vi "Embedded UI.TestLauncher.vi"() -> ()   [LabVIEW 2019, in "Embedded UI.lvclass"]
doc: "JKI State Machine Objects (SMO) 1.0.0.5\nJKI - JKI\nCopyright (c) 2016, JKI"
uses:
  Embedded UI.lvclass
  <vilib>/JKI/JKI SMO/SMO/SMO.lvclass
  <vilib>/JKI/JKI SMO/SMO.UI/SMO.UI.lvclass
  <vilib>/JKI/JKI SMO/SMO/Typedefs/SMOState --Enum.ctl
  C:/Program Files (x86)/National Instruments/LabVIEW 2019/vi.lib/JKI/JKI SMO/SMO.UI/SMO.UI.lvclass
  C:/Program Files (x86)/National Instruments/LabVIEW 2019/vi.lib/JKI/JKI SMO/SMO/SMO.lvclass
panel:
  in  "Change Name":bool
  out "Get Name":string
  in  "Set Name":string
  in  "Embed?":bool
  out "error out":errorcluster
  in  "Stop":bool
  # "SMO UI Test Launcher"
  # "For instructions on how to use the JKI State Machine Objects, examples and video tutorials, visit:\nhttp://jki.net/state-machine-objects/\n\nJKI State Machine Objects™\nhttp://jki.net/state-machine-objects/\nCopyright (C) 2005-2015, JKI <info@jki.net>\nALL RIGHTS RESERVED"
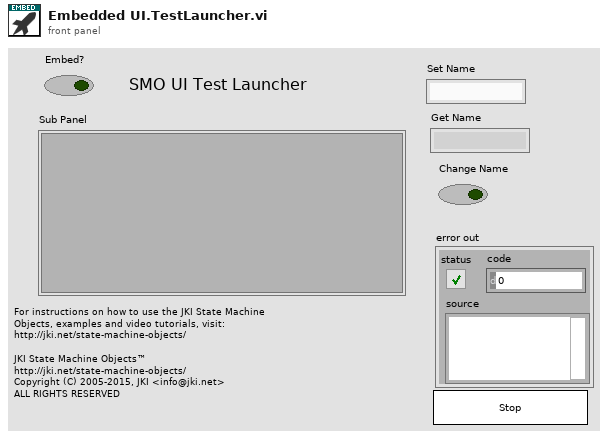
[diagram p1: front panel]
types:
  T1 = typedef "SMO.lvclass/Public Events.ctl" = cluster{"Error":refnum<user-event>, "State":refnum<user-event>, "Reserve State":refnum<user-event>}
  T2 = typedef "SMO.UI.lvclass/PublicEvents--Cluster.ctl" = cluster{"UI Hidden":refnum<user-event>, "UI State":refnum<user-event>}
  T3 = typedef "SMO.lvclass/SMOState --Enum.ctl" = enum16{"unknown", "Created", "Started", "Stopped"}
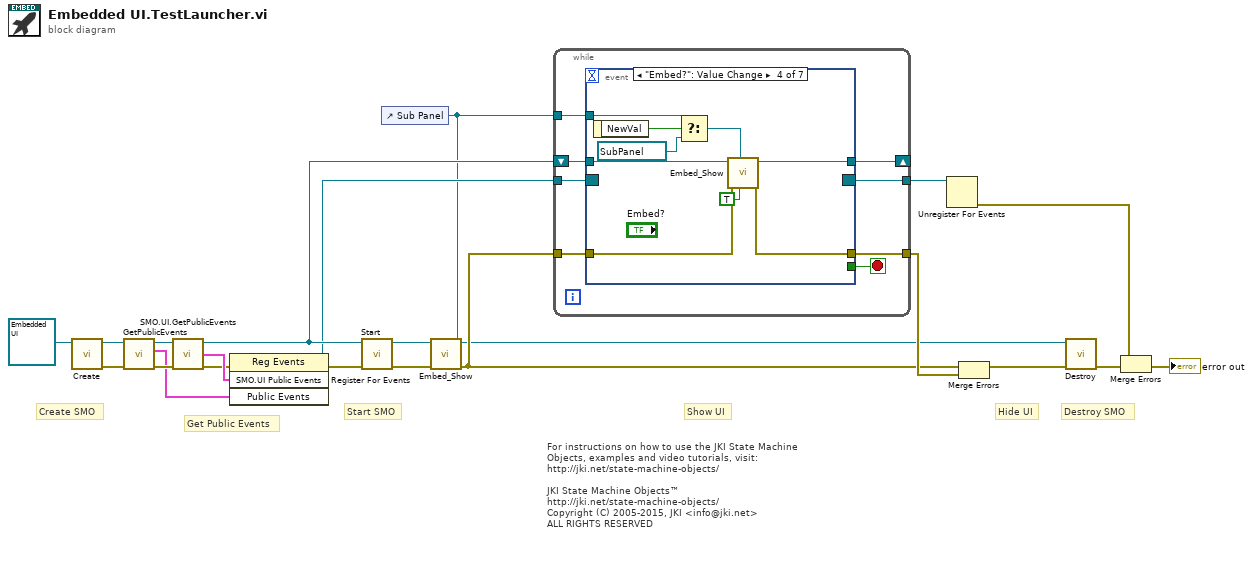
[diagram p0: block diagram]
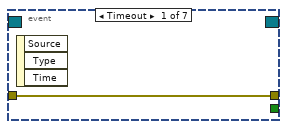
[diagram p2: hidden frame]
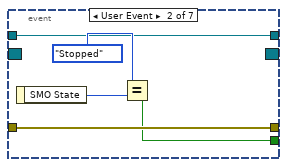
[diagram p3: hidden frame]
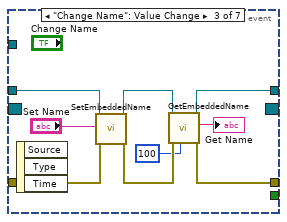
[diagram p4: hidden frame]
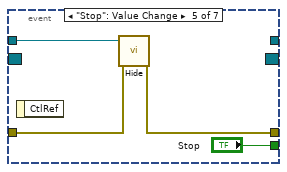
[diagram p5: hidden frame]
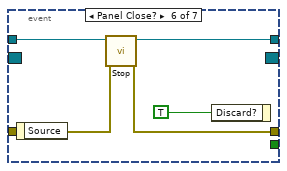
[diagram p6: hidden frame]
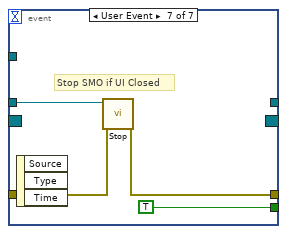
[diagram p7: hidden frame]
diagram:
  # "Hide UI"
  # "Show UI"
  # "For instructions on how to use the JKI State Machine Objects, examples and video tutorials, visit:\nhttp://jki.net/state-machine-objects/\n\nJKI State Machine Objects™\nhttp://jki.net/state-machine-objects/\nCopyright (C) 2005-2015, JKI <info@jki.net>\nALL RIGHTS RESERVED"
  # "Get Public Events"
  # "Start SMO"
  # "Destroy SMO"
  # "Create SMO"
  n1 = call <vilib>:"Create.vi"("SMO"=refnum<class "Embedded UI.lvclass"> refnum ("SMO.Template.lvclass")) -> ("error out"=w10:errorcluster, "SMO out"=w9:refnum<class "Embedded UI.lvclass">)  [unwired: 8 in, 1 out]
  n2 = call <vilib>:"GetPublicEvents.vi"("error in (no error)"=w10, "SMO"=w9) -> ("error out"=w7:errorcluster, "Public Events"=w6:T1, "SMO out"=w8:refnum<class "Embedded UI.lvclass">)  [unwired: 7 in]
  n3 = call <vilib>:"SMO.UI.GetPublicEvents.vi"("error in (no error)"=w7, "SMO.UI"=w8) -> ("error out"=w13:errorcluster, "SMO.UI Public Events"=w14:T2, "SMO.UI out"=w15:refnum<class "Embedded UI.lvclass">)  [unwired: 7 in]
  n4 = register-events(error in=w13, w14, w6) -> (reference out=w11:refnum<event-registration>, error out=w12:errorcluster)  [unwired: 1 in]
  n5 = call <vilib>:"Start.vi"("error in (no error)"=w12, "SMO"=w15) -> ("error out"=w5:errorcluster, "SMO out"=w3:refnum<class "Embedded UI.lvclass">)  [unwired: 8 in]
  n6 = control-ref of="Sub Panel"() -> (w1:refnum<vi>)
  n7 = call "Embed_Show.vi"("Sub Panel"=w1, "error in (no error)"=w5, "EmbeddedSMO in"=w3) -> ("error out"=w4:errorcluster, "EmbeddedSMO out"=w2:refnum<class "Embedded UI.lvclass">)  [unwired: 7 in]
  n8 = while {
    tunnel: w11 -> [w27]
    tunnel: [w26] -> w22
    tunnel: w1 -> [w24]
    shift-right: [w23] -> _
    shift-left: w15 -> [w25]
    tunnel: w4 -> [w28]
    tunnel: [w29] -> w21
    stop <- w30 stop-if-true
    n9 = event shown="[3] \"Embed?\": Value Change" {
      selector: w27 -> [_ _ _ _ _ _ _]
      dyn-events: [_ _ _ _ _ _ _] -> w26
      timeout: _ -> [_ _ _ _ _ _ _]
      tunnel: [_ w33 _ _ "Stop" _ TRUE ("OK")] -> w30
      tunnel: w25 -> [_ w32 w45 w52 w58 w62 w67]
      tunnel: [w31 w36 w39 w50 w55 w60 w66] -> w29
      tunnel: w28 -> [w31 w36 w43 w51 w57 w61 w65]
      tunnel: w24 -> [_ _ _ w54 _ _ _]
      tunnel: [_ w32 w41 w47 _ w59 _] -> w23
      event Timeout {
        n10 = event-data() -> ()  [unwired: 1 in, 3 out]
      }
      event User Event {
        n11 = event-data() -> ("SMO State"=w35:T3)  [unwired: 1 in]
        n12 = Equal?(x=SMOState_--Enum."Stopped", y=w35) -> (x = y?=w33:bool)
      }
      event "Change Name": Value Change {
        n13 = event-data() -> ()  [unwired: 1 in, 3 out]
        n14 = call "SetEmbeddedName.vi"("error in (no error)"=w43, "Name"="Set Name", "EmbeddedSMO in"=w45) -> ("error out"=w40:errorcluster, "EmbeddedSMO out"=w42:refnum<class "Embedded UI.lvclass">)  [unwired: 7 in]
        n15 = call "GetEmbeddedName.vi"("timeout in ms (-1)"=100, "error in (no error)"=w40, "EmbeddedSMO in"=w42) -> ("error out"=w39:errorcluster, "Name"=→"Get Name":string, "EmbeddedSMO out"=w41:refnum<class "Embedded UI.lvclass">)  [unwired: 6 in]
      }
      event "Embed?": Value Change {
        n16 = event-data() -> ("NewVal"=w53:bool)  [unwired: 1 in]
        n17 = Select(t=w54, s=w53, f=refnum<vi> refnum) -> (s? t:f=w49:refnum<vi>)
        n18 = call "Embed_Show.vi"("Force?"=TRUE, "Sub Panel"=w49, "error in (no error)"=w51, "EmbeddedSMO in"=w52) -> ("error out"=w50:errorcluster, "EmbeddedSMO out"=w47:refnum<class "Embedded UI.lvclass">)  [unwired: 6 in]
      }
      event "Stop": Value Change {
        n19 = event-data() -> ()  [unwired: 1 in, 1 out]
        n20 = call <vilib>:"Hide.vi"("error in (no error)"=w57, "SMO.UI"=w58) -> ("error out"=w55:errorcluster)  [unwired: 8 in, 1 out]
      }
      event Panel Close? {
        n21 = event-data() -> ()  [unwired: 1 in, 1 out]
        n22 = call <vilib>:"Stop.vi"("error in (no error)"=w61, "SMO"=w62) -> ("error out"=w60:errorcluster, "SMO out"=w59:refnum<class "Embedded UI.lvclass">)  [unwired: 8 in]
        n23 = event-data("Discard?"=TRUE ("OK")) -> ()  [unwired: 1 in, 1 out]
      }
      event User Event {
        # "Stop SMO if UI Closed"
        n24 = event-data() -> ()  [unwired: 1 in, 3 out]
        n25 = call <vilib>:"Stop.vi"("error in (no error)"=w65, "SMO"=w67) -> ("error out"=w66:errorcluster)  [unwired: 8 in, 1 out]
      }
    }
  }
  n26 = Unregister For Events(event registration refnum=w22) -> (error out=w20:errorcluster)  [unwired: 1 in]
  n27 = Merge Errors(w4, w21) -> (w16:errorcluster)
  n28 = call <vilib>:"Destroy.vi"("error in (no error)"=w16, "SMO"=w2) -> ("error out"=w18:errorcluster)  [unwired: 9 in]
  n29 = Merge Errors(w20, w18) -> (→"error out":errorcluster)
